vi "Debug_WFS_Tilt.vi"() -> ()   [LabVIEW 2010]
uses:
  <vilib>/userdefined/High Color/nirio_resource_hc.ctl
  AODAcq/AODAcq.lvclass
  <vilib>/userDefined/High Color/IMAQdx.ctl
  <vilib>/vision/driver/IMAQdx.llb/IMAQdx Camera Control Mode.ctl
  <vilib>/rvi/interface/nirviReadWriteControl/nirviReadWriteControl.xnode
  FPGA_Control/AODRef.ctl
  FPGA_Control/FPGA Bitfiles/AODControl_FPGATarget_5751Acquire_1926D8C3.lvbitx
  FPGA_Control/AOD Control (FPGA).vi
  <vilib>/DAQmx/write.llb/DAQmx Write (Analog DBL 1Chan 1Samp).vi
  <vilib>/DAQmx/read.llb/DAQmx Read (Analog 1D DBL NChan 1Samp).vi
  <vilib>/DAQmx/create/channels.llb/DAQmx Create Channel (AI-Voltage-Basic).vi
  <vilib>/daqmx/miscellaneous.llb/DAQmx Fill In Error Info.vi
  <vilib>/Utility/file.llb/Write To Spreadsheet File (DBL).vi
  <vilib>/vision/driver/NI_Vision_Acquisition_Software.lvlib
panel:
  in  "Reps":i32=1
  out "Image":T1(plugin-control)
  in  "Measure centroid":bool
  out "Power":dbl
  in  "Save":bool
  in  "Range":dbl=214748364.8
  in  "stop":bool
  out "Corodinate Num":i32
  out "Num Coordinates":i32
  in  "NYHP":i32=10
  in  "NYLP":i32=10
  in  "NXHP":i32=10
  in  "NXLP":i32=10
  in  "Measure WFS":bool
  in  "Measure Power":bool
  in  "Hold time (ms)":u32=500
  in  "RIO Device":T2="RIO0"
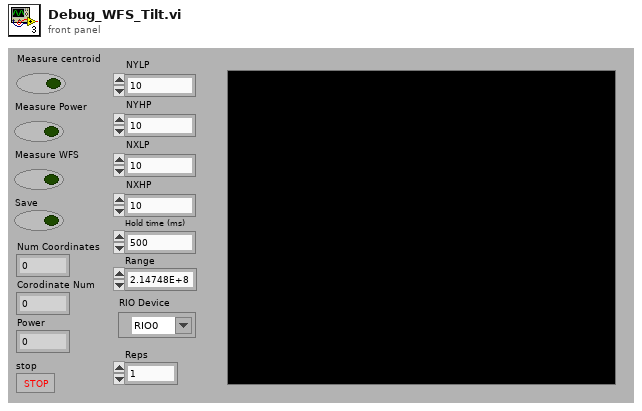
[diagram p1: front panel]
types:
  T1 = typedef "IMAQ Image.ctl" = refnum<image>
  T2 = typedef "nirio_resource_hc.ctl" = tag
  T3 = typedef "NI_Vision_Acquisition_Software.lvlib/IMAQdx Camera Control Mode.ctl" = enum32{"Controller", "Listener"}
  T4 = typedef "IMAQdx.ctl" = refnum<k21>
  T5 = typedef "Image Type" = u32
  T6 = enum16{"Read", "Write", "ReadWrite", "BufferedRead", "BufferedReadWrite"}
  T7 = cluster{"XHP":i32, "XLP":i32, "YHP":i32, "YLP":i32}[]
  T8 = typedef "AODRef.ctl" = refnum<k20>
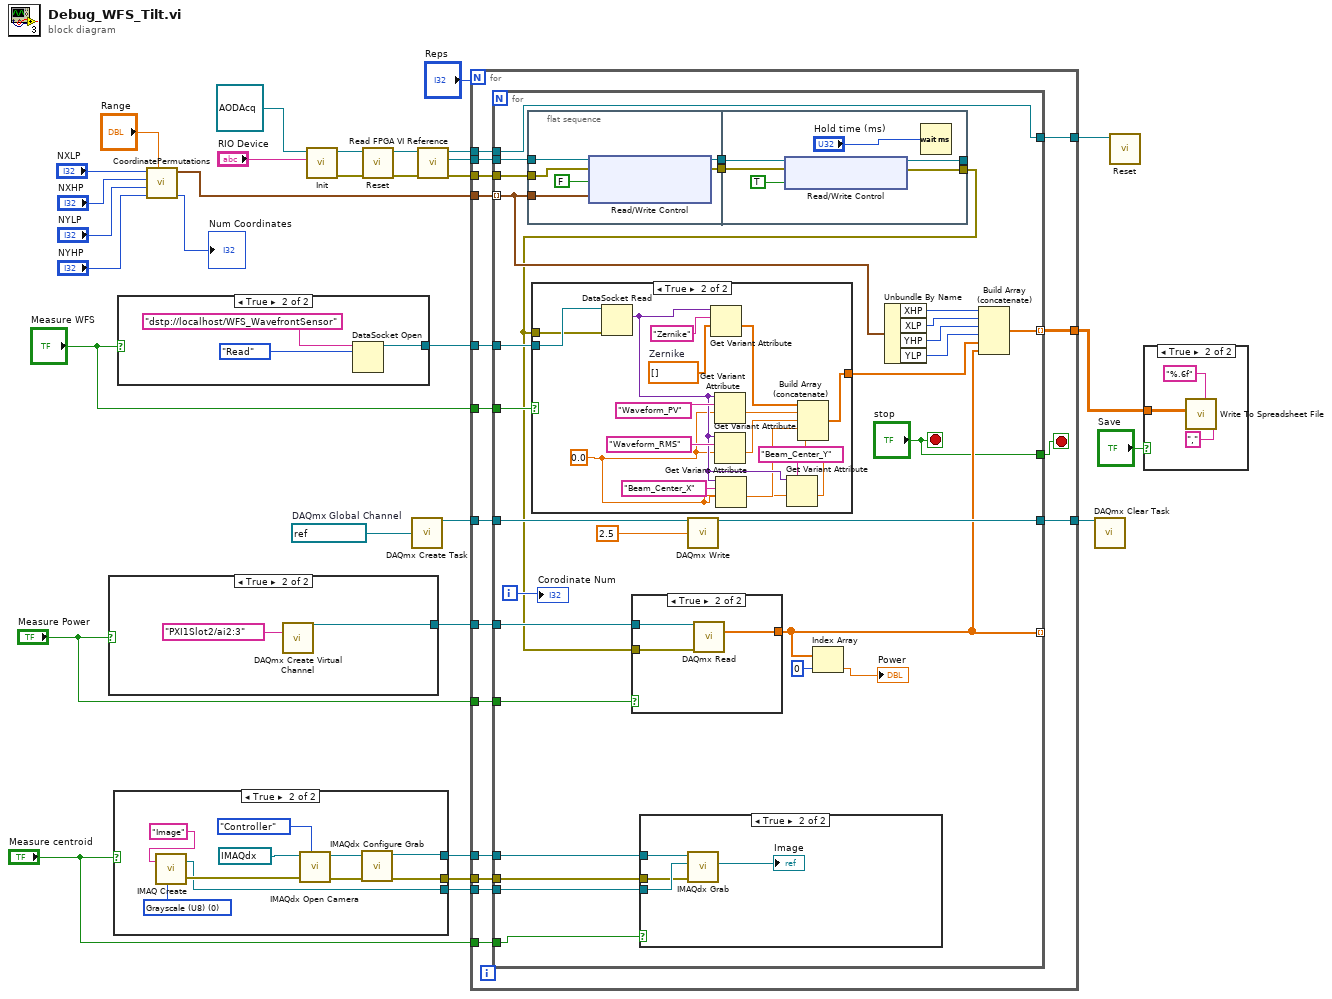
[diagram p0: block diagram]
diagram:
  w21 = refnum<k21> "AOD Gain"  # DAQmx Global Channel
  n1 = case shown="True" "Measure Power" {
    tunnel: [_ w32] -> w9
    frame False {
    }
    frame True {
      n2 = call-poly <vilib>:"DAQmx Create Virtual Channel.vi"("physical channels"=tag "PXI1Slot2/ai2:3") -> ("task out"=w32:refnum<k21>)  [unwired: 13 in, 1 out]
    }
  }
  n3 = case shown="True" "Measure centroid" {
    tunnel: [_ w35] -> w7
    tunnel: [_ w39] -> w5
    tunnel: [_ w34] -> w4
    frame False {
    }
    frame True {
      w41 = T5 0 items=["Grayscale (U8)", "Grayscale (I16)", "Grayscale (SGL)", "Complex (CSG)", "RGB (U32)", "HSL (U32)", "RGB (U64)", "Grayscale (U16)"] ("Image Type")
      n4 = call "IMAQ Create"("Image Name"="Image", "Image Type"=w41) -> ("New Image"=w39:T1, "error out"=w40:errorcluster)  [unwired: 3 in]
      n5 = call <vilib>:"IMAQdx Open Camera.vi"("Camera Control Mode"=IMAQdx_Camera_Control_Mode."Controller", "error in"=w40, "Session In"=T4 "cam1") -> ("error out"=w37:errorcluster, "Session Out"=w36:T4)  [unwired: 7 in]
      n6 = call <vilib>:"IMAQdx Configure Grab.vi"("error in"=w37, "Session In"=w36) -> ("error out"=w34:errorcluster, "Session Out"=w35:T4)  [unwired: 8 in]
    }
  }
  n7 = case shown="True" "Measure WFS" {
    tunnel: [_ w44] -> w22
    frame False {
    }
    frame True {
      n8 = DataSocket Open(10:T6."Read" ("mode"), 11:"dstp://localhost/WFS_WavefrontSensor" ("URL")) -> (3:w44:refnum<k13>)  [unwired: 2 in, 1 out]
    }
  }
  n9 = call "CoordinatePermutations.vi"("Range"="Range", "NYHP"="NYHP", "NYLP"="NYLP", "NXHP"="NXHP", "NXLP"="NXLP") -> ("Num Coordinates"=→"Num Coordinates":i32, "Coordinates"=w3:T7)  [unwired: 5 in]
  n10 = call "Init.vi"("RIO Device"="RIO Device", "AODAcq in"=refnum<class "AODAcq.lvclass"> refnum ("AODAcq.lvclass")) -> ("error out"=w28:errorcluster, "AODAcq out"=w29:refnum<class "AODAcq.lvclass">)  [unwired: 8 in]
  n11 = call-dynamic "Reset.vi"("error in (no error)"=w28, "AODAcq in"=w29) -> ("error out"=w25:errorcluster, "AODAcq out"=w27:refnum<class "AODAcq.lvclass">)  [unwired: 8 in]
  n12 = call <vilib>:"DAQmx Create Task.vi"("global virtual channels"=w21) -> ("task out"=w20:refnum<k21>)  [unwired: 4 in, 10 out]
  n13 = call-dynamic "Read FPGA VI Reference.vi"("error in (no error)"=w25, "AODAcq in"=w27) -> ("error out"=w24:errorcluster, "FPGA VI Reference"=w26:T8, "AODAcq out"=w18:refnum<class "AODAcq.lvclass">)  [unwired: 7 in]
  n14 = for {
    N: "Reps" -> [_]
    tunnel: w26 -> [w63]
    tunnel: w24 -> [w62]
    tunnel: "Measure WFS" -> [w61]
    tunnel: w22 -> [w60]
    tunnel: w20 -> [w59]
    tunnel: [w58] -> w19
    tunnel: w18 -> [w57]
    tunnel: [w56] -> w1
    tunnel: [w55] -> w11
    tunnel: w9 -> [w54]
    tunnel: "Measure Power" -> [w53]
    tunnel: w7 -> [w52]
    tunnel: "Measure centroid" -> [w51]
    tunnel: w5 -> [w50]
    tunnel: w4 -> [w49]
    tunnel: w3 -> [w48]
    stop <- w47 stop-if-true
    n15 = for {
      tunnel: w63 -> [w91]
      tunnel: w48 -> [w81] mode=indexing
      tunnel: w62 -> [w89]
      tunnel: w61 -> [w88]
      tunnel: w60 -> [w87]
      tunnel: w59 -> [w86]
      tunnel: [w84] -> w58
      tunnel: w57 -> [w83]
      tunnel: [w83] -> w56
      tunnel: [w75] -> w55 mode=indexing
      tunnel: w54 -> [w74]
      tunnel: w53 -> [w72]
      tunnel: [w71] -> _ mode=indexing
      tunnel: w52 -> [w67]
      tunnel: w51 -> [w68]
      tunnel: w50 -> [w66]
      tunnel: w49 -> [w65]
      tunnel: ["stop"] -> w47
      i -> [w82]
      stop <- "stop" stop-if-true
      n16 = flat-sequence {
        tunnel: w91 -> [w121]
        tunnel: [w119] -> w92
        tunnel: w81 -> [w118]
        tunnel: [w117] -> w90
        tunnel: w89 -> [w116]
        tunnel: w92 -> [w144]
        tunnel: w90 -> [w141]
        tunnel: [w140] -> w73
        tunnel: [w139] -> _
        frame #0 {
          n17 = xnode "Read/Write Control"("FPGA VI Reference In"=w121, "error in"=w116, "Debug.SetCoordinate"=FALSE, "Debug.Coordinate"=w118) -> ("FPGA VI Reference Out"=w119:T8, "error out"=w117:errorcluster)
        }
        frame #1 {
          n18 = xnode "Read/Write Control"("FPGA VI Reference In"=w144, "error in"=w141, "Debug.SetCoordinate"=TRUE) -> ("FPGA VI Reference Out"=w139:T8, "error out"=w140:errorcluster)
          n19 = Wait (ms)(milliseconds to wait="Hold time (ms)") -> ()  [unwired: 1 out]
        }
      }
      n20 = case shown="True" w88 {
        tunnel: w87 -> [_ w113]
        tunnel: w73 -> [_ w112]
        tunnel: [_ w106] -> w76
        frame False {
        }
        frame True {
          w101 = 0.0
          w115 = dbl[] []  # Zernike
          n21 = DataSocket Read(8:w112, 11:w113) -> (2:w105:variant)  [unwired: 3 in, 6 out]
          n22 = Get Variant Attribute(Variant=w105, name="Zernike", default value (empty Variant)=w115) -> (value=w109:dbl[])  [unwired: 1 in, 3 out]
          n23 = Get Variant Attribute(Variant=w105, name="Waveform_PV", default value (empty Variant)=w101) -> (value=w108:dbl)  [unwired: 1 in, 3 out]
          n24 = Get Variant Attribute(Variant=w105, name="Waveform_RMS", default value (empty Variant)=w101) -> (value=w107:dbl)  [unwired: 1 in, 3 out]
          n25 = Get Variant Attribute(Variant=w105, name="Beam_Center_X", default value (empty Variant)=w101) -> (value=w102:dbl)  [unwired: 1 in, 3 out]
          n26 = Get Variant Attribute(Variant=w105, name="Beam_Center_Y", default value (empty Variant)=w101) -> (value=w100:dbl)  [unwired: 1 in, 3 out]
          n27 = Build Array (concatenate)(w109, w108, w107, w102, w100) -> (w106:dbl[])
        }
      }
      n28 = case shown="True" w72 {
        tunnel: w74 -> [_ w99]
        tunnel: w73 -> [_ w98]
        tunnel: [_ w97] -> w71
        frame False {
        }
        frame True {
          n29 = call-poly <vilib>:"DAQmx Read.vi"("task/channels in"=w99, "error in"=w98) -> ("data"=w97:dbl[])  [unwired: 11 in, 2 out]
        }
      }
      n30 = case shown="True" w68 {
        tunnel: w67 -> [_ w96]
        tunnel: w66 -> [_ w94]
        tunnel: w65 -> [_ w93]
        frame False {
        }
        frame True {
          n31 = call <vilib>:"IMAQdx Grab.vi"("error in"=w93, "Image In"=w94, "Session In"=w96) -> ("Image Out"=→"Image":T1)  [unwired: 5 in, 3 out]
        }
      }
      n32 = call-poly <vilib>:"DAQmx Write.vi"("task/channels in"=w86, "data"=2.5) -> ("task out"=w84:refnum<k21>)  [unwired: 11 in, 2 out]
      n33 = Index Array(array=w71, index=0) -> (element=→"Power":dbl)
      n34 = Unbundle By Name(w81) -> ("XHP"=w80:i32, "XLP"=w79:i32, "YHP"=w78:i32, "YLP"=w77:i32)
      n35 = Build Array (concatenate)(w80, w79, w78, w77, w76, w71) -> (w75:dbl[])
      "Corodinate Num" <- w82
    }
  }
  n36 = call <vilib>:"DAQmx Clear Task.vi"("task in"=w19) -> ()  [unwired: 14 in, 1 out]
  n37 = call-dynamic "Reset.vi"("AODAcq in"=w1) -> ()  [unwired: 9 in, 2 out]
  n38 = case shown="True" "Save" {
    tunnel: w11 -> [_ w160]
    frame False {
    }
    frame True {
      n39 = call-poly <vilib>:"Write To Spreadsheet File.vi"("delimiter (\\t)"="," ("delimiter (\\t)"), "format (%.3f)"="%.6f", "2D data"=w160) -> ()  [unwired: 5 in, 1 out]
    }
  }
